vi "Microscopy.Detect Trigger Edge.vi"(6 "Ready for Next Record?":bool, 7 "Trigger Type":T2(ring)=enum."Software Trigger", 8 "Data Valid In":bool, 9 "Software Trigger from Host":bool, 10 "Digita IO Trigger":bool, 11 "Analog Channel Data":i16[](array[numeric])=[0, 0, 0, 0]) -> (0 "Data Valid Out":bool, 1 "Reference Trigger Edge?":bool, 3 "Analog Channel Data":T1, 4 "Trig Offset":u8)   [LabVIEW 2012]
doc: "This VI detects rising edge on a select trigger Type.\n\nThe trigger type is selected from the Host. The trigger types can be\n1) External Digital Trigger\n2) Software Trigger from Host\n3) Immediate Trigger"
uses:
  Multi-Channel Analog Input Data.ctl
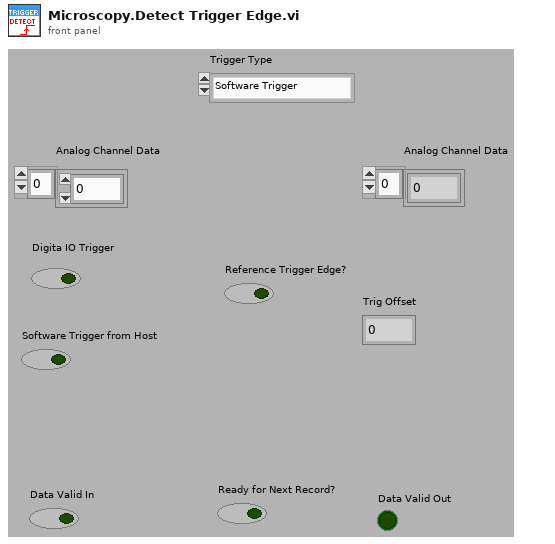
[diagram p1: front panel]
types:
  T1 = typedef "Multi-Channel Analog Input Data.ctl" = i16[]
  T2 = enum8{"External Digital Trigger", "Software Trigger", "Immediate Trigger"}
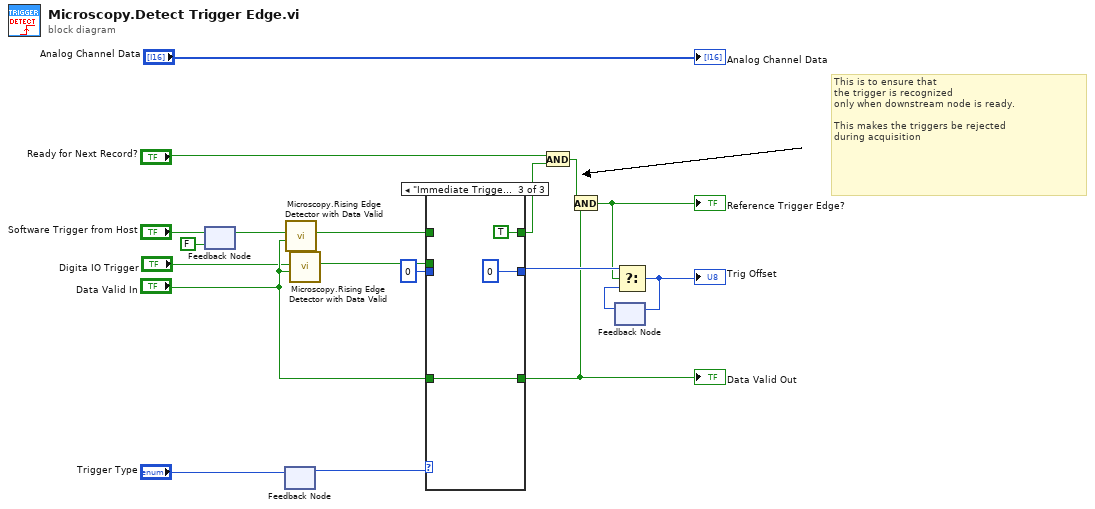
[diagram p0: block diagram]
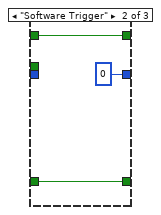
[diagram p3: hidden frame]
diagram:
  # "This is to ensure that\nthe trigger is recognized\nonly when downstream node is ready.\n\nThis makes the triggers be rejected\nduring acquisition"
  n1 = feedback-in #1("Software Trigger from Host") -> ()
  n2 = feedback #1(FALSE ("Software Trigger from Host")) -> (w9:bool)
  n3 = feedback #2() -> (w18:T2)  [unwired: 1 in]
  n4 = feedback-in #2("Trigger Type") -> ()
  n5 = call "Microscopy.Rising Edge Detector with Data Valid.vi"("Data Valid"="Data Valid In", "signal"=w9) -> ("edge detected"=w11:bool)  [unwired: 9 in]
  n6 = call "Microscopy.Rising Edge Detector with Data Valid.vi"("Data Valid"="Data Valid In", "signal"="Digita IO Trigger") -> ("edge detected"=w2:bool)  [unwired: 9 in]
  n7 = case shown="\"Immediate Trigger\"" w18 {
    tunnel: [w22 u8 0 ("Trig Offset") u8 0 ("Trig Offset")] -> w14
    tunnel: u8 0 ("Trig Offset") -> [w22 _ _]
    tunnel: w2 -> [w21 _ _]
    tunnel: [w21 w25 TRUE ("edge detected")] -> w15
    tunnel: w11 -> [_ w25 _]
    tunnel: "Data Valid In" -> [w20 w23 w27]
    tunnel: [w20 w23 w27] -> w7
    frame "External Digital Trigger", Default {
    }
    frame "Software Trigger" {
    }
    frame "Immediate Trigger" {
    }
  }
  "Data Valid Out" <- w7
  n8 = And(x="Ready for Next Record?", y=w15) -> (x .and. y?=w6:bool)
  n9 = And(x=w6, y=w7) -> (x .and. y?=w5:bool)
  "Reference Trigger Edge?" <- w5
  n10 = feedback #3() -> (w13:u8)  [unwired: 1 in]
  n11 = Select(t=w14, s=w5, f=w13) -> (s? t:f=w12:u8)
  "Trig Offset" <- w12
  n12 = feedback-in #3(w12) -> ()
  "Analog Channel Data" <- "Analog Channel Data"
